vi "Test Clean Children List.vi"(8 "error in (no error)":errorcluster) -> (0 "error out":errorcluster)   [LabVIEW 2017, in "Unit Tests.lvlib"]
uses:
  Unit Tests.lvlib
  source/Browser Core/Server Classes/Base Tree/Base Tree.lvclass
  source/Browser Core/Node Classes/Generic Node/Generic Node.lvclass
  source/Browser Core/Node Classes/Generic Node/Generic Node.lvclass/Generic Node.ctl
  <vilib>/addons/_JKI Toolkits/Caraya/classes/Test/Test.lvclass
  <vilib>/addons/_JKI Toolkits/Caraya/classes/Assert/Assert.lvclass
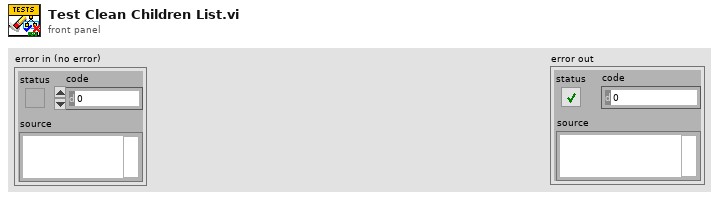
[diagram p1: front panel]
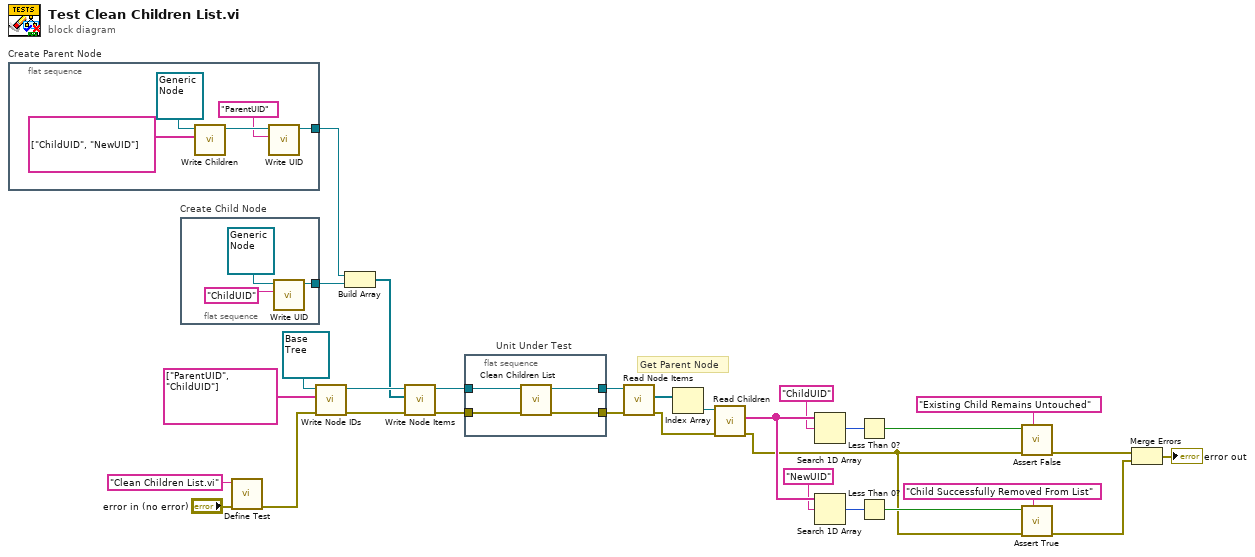
[diagram p0: block diagram]
diagram:
  # "Get Parent Node"
  n1 = flat-sequence "Create Parent Node" {
    tunnel: [w31] -> w25
    frame #0 {
      n2 = call "Write Children.vi"("Children"=string[] ["ChildUID", "NewUID"], "Generic Node in"=refnum<class "Generic Node.lvclass"> refnum ("Class Node")) -> ("Generic Node out"=w33:refnum<class "Generic Node.lvclass">)  [unwired: 8 in, 1 out]
      n3 = call "Write UID.vi"("UID"="ParentUID", "Generic Node in"=w33) -> ("Generic Node out"=w31:refnum<class "Generic Node.lvclass">)  [unwired: 8 in, 1 out]
    }
  }
  n4 = flat-sequence "Create Child Node" {
    tunnel: [w36] -> w26
    frame #0 {
      n5 = call "Write UID.vi"("UID"="ChildUID", "Generic Node in"=refnum<class "Generic Node.lvclass"> refnum ("Class Node")) -> ("Generic Node out"=w36:refnum<class "Generic Node.lvclass">)  [unwired: 8 in, 1 out]
    }
  }
  n6 = call <vilib>:"Define Test.vi"("error in (no error)"="error in (no error)", "Label (VI Title)"="Clean Children List.vi") -> ("error out"=w22:errorcluster)  [unwired: 9 in]
  n7 = call "Write Node IDs.vi"("error in (no error)"=w22, "Node IDs"=string[] ["ParentUID", "ChildUID"], "Base Tree in"=refnum<class "Base Tree.lvclass"> refnum) -> ("error out"=w21:errorcluster, "Base Tree out"=w24:refnum<class "Base Tree.lvclass">)  [unwired: 7 in]
  n8 = Build Array(w25, w26) -> (w23:refnum<class "Generic Node.lvclass">[])
  n9 = call "Write Node Items.vi"("error in (no error)"=w21, "Node Items"=w23, "Base Tree in"=w24) -> ("error out"=w19:errorcluster, "Base Tree out"=w20:refnum<class "Base Tree.lvclass">)  [unwired: 7 in]
  n10 = flat-sequence "Unit Under Test" {
    tunnel: w20 -> [w42]
    tunnel: w19 -> [w41]
    tunnel: [w40] -> w18
    tunnel: [w39] -> w17
    frame #0 {
      n11 = call "Clean Children List.vi"("error in (no error)"=w41, "Base Tree in"=w42) -> ("error out"=w39:errorcluster, "Base Tree out"=w40:refnum<class "Base Tree.lvclass">)  [unwired: 8 in]
    }
  }
  n12 = call "Read Node Items.vi"("error in (no error)"=w17, "Base Tree in"=w18) -> ("error out"=w14:errorcluster, "Node Items"=w16:refnum<class "Generic Node.lvclass">[])  [unwired: 7 in, 1 out]
  n13 = Index Array(array=w16) -> (element=w15:refnum<class "Generic Node.lvclass">)  [unwired: 1 in]
  n14 = call "Read Children.vi"("error in (no error)"=w14, "Generic Node in"=w15) -> ("error out"=w6:errorcluster, "Children"=w13:string[])  [unwired: 7 in, 1 out]
  n15 = Search 1D Array(1D array=w13, element="ChildUID") -> (index of element=w10:i32)  [unwired: 1 in]
  n16 = Search 1D Array(1D array=w13, element="NewUID") -> (index of element=w9:i32)  [unwired: 1 in]
  n17 = Less Than 0?(x=w10) -> (x < 0?=w7:bool)
  n18 = Less Than 0?(x=w9) -> (x < 0?=w8:bool)
  n19 = call <vilib>:"Assert False.vi"("Label"="Existing Child Remains Untouched" ("Label (VI Title)"), "error in (no error)"=w6, "False?"=w7) -> ("error out"=w5:errorcluster)  [unwired: 8 in]
  n20 = call <vilib>:"Assert True.vi"("Label"="Child Successfully Removed From List" ("Label (VI Title)"), "error in (no error)"=w6, "True?"=w8) -> ("error out"=w4:errorcluster)  [unwired: 8 in]
  n21 = Merge Errors(w5, w4) -> (→"error out":errorcluster)
